vi "Device Manager.vi"() -> ()   [LabVIEW 2026]
doc: "This template is for the Queued Message Handler design pattern.\n\nThe Event Handling Loop generates messages based on user interface actions.\n\nThe Message Handling Loop processes messages generated by the Event Handling Loop, or by other messages. The messages are string values, so new messages can be added easily to the Message Cases case structure in the Message Handling Loop. Each message cluster can also provide an optional value for Message Data, which is a variant that can be converted to whatever message-specific data is required."
uses:
  controls/Device Manager Private Data.ctl
  support/Message Queue/Enqueue Message (Single).vi
  <vilib>/Utility/error.llb/Error Cluster From Error Code.vi
  <vilib>/ErrorRing/Error Ring.xnode
  support/Message Queue/Message Queue.lvlib
  support/User Event - Stop/User Event - Stop.lvlib
panel:
  in  "Exit":bool
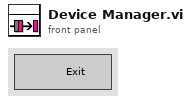
[diagram p1: front panel]
types:
  T1 = typedef "Device Manager Private Data.ctl" = cluster{"Exit Button Ref":refnum<vi>}
  T2 = typedef "Message Queue.lvlib/All Message Queues.ctl" = cluster{"Device Manager":refnum<queue>, "Front Panel Emulator":refnum<queue>, "Servo Motor Emulator":refnum<queue>}
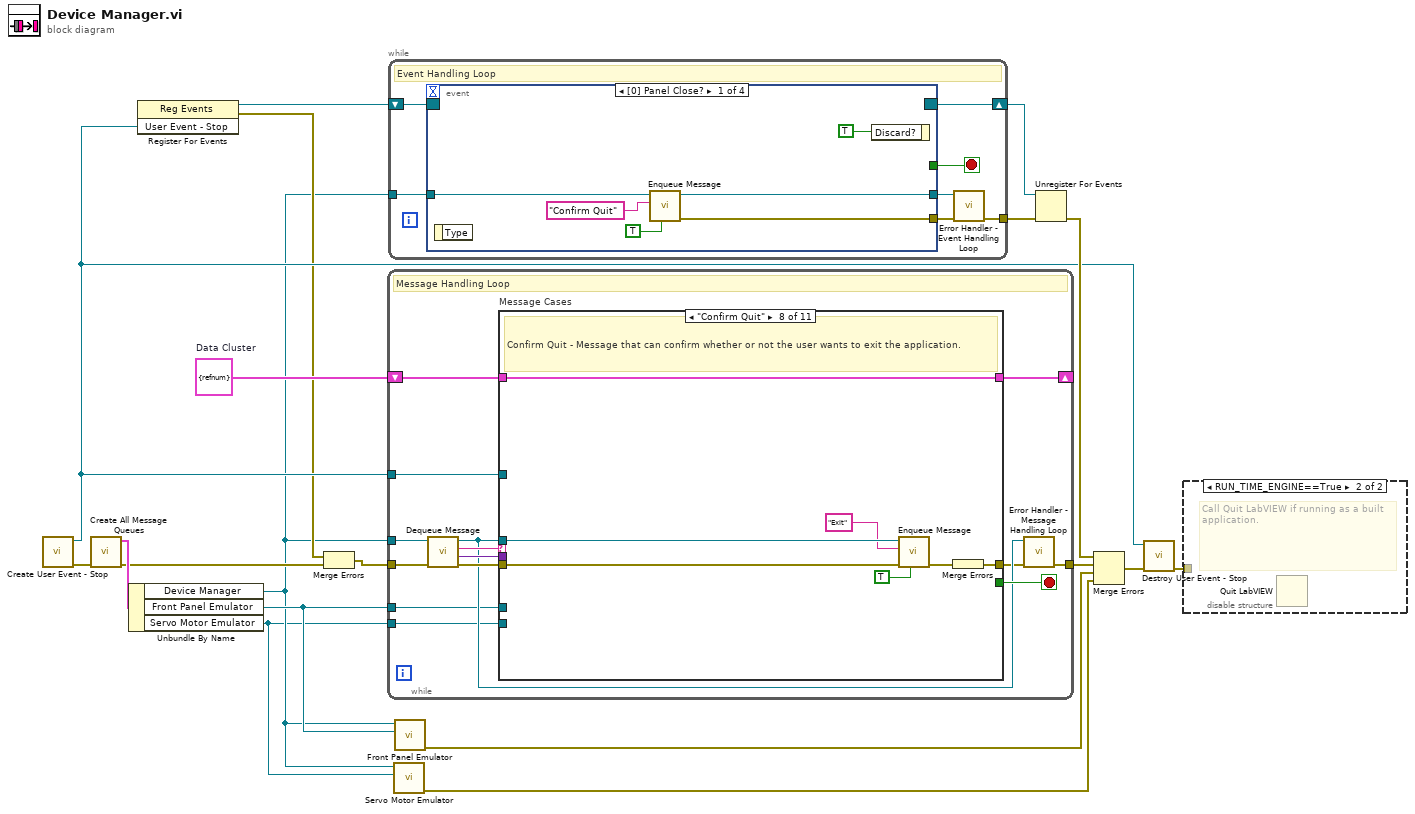
[diagram p0: block diagram]
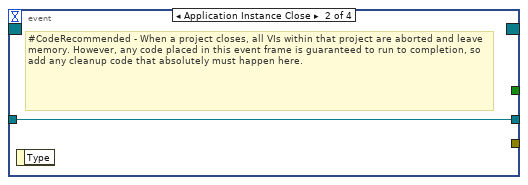
[diagram p3: hidden frame]
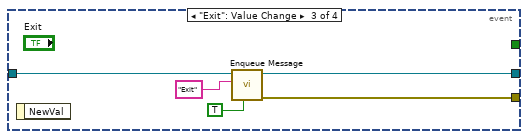
[diagram p4: hidden frame]
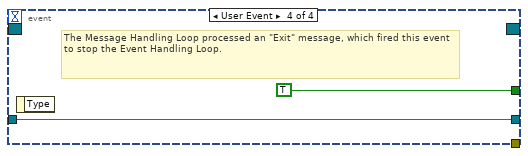
[diagram p5: hidden frame]
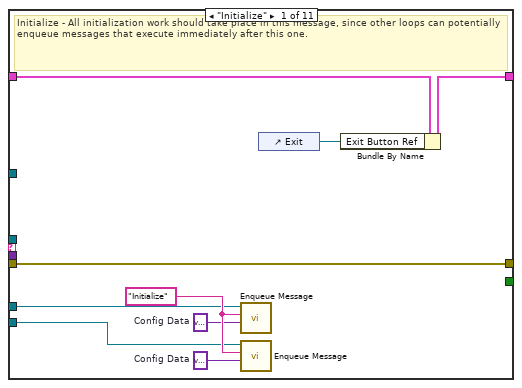
[diagram p6: hidden frame]
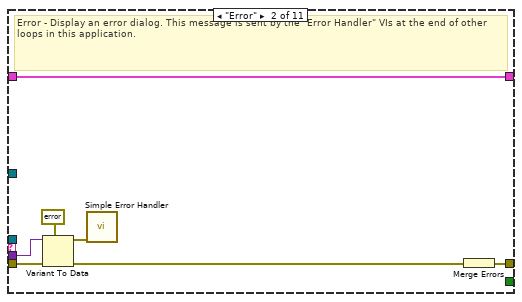
[diagram p7: hidden frame]
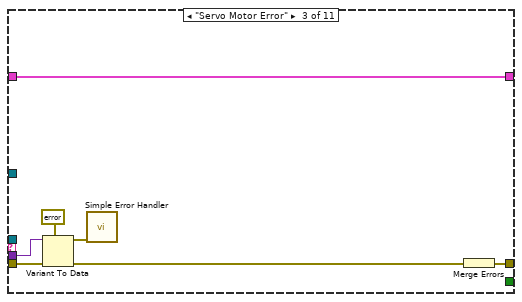
[diagram p8: hidden frame]
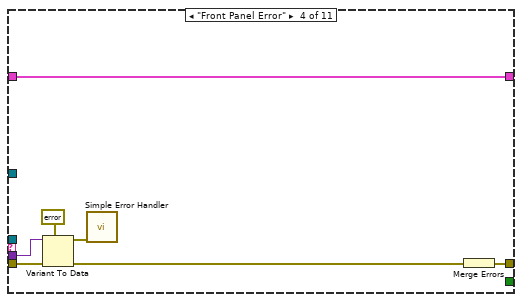
[diagram p9: hidden frame]
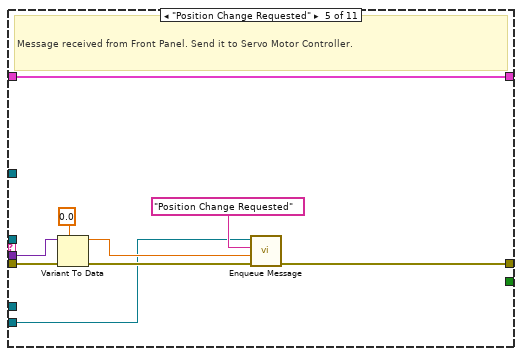
[diagram p10: hidden frame]
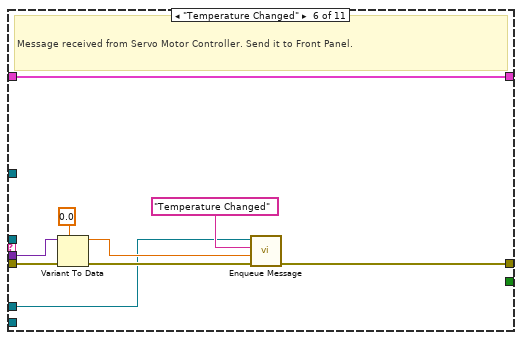
[diagram p11: hidden frame]
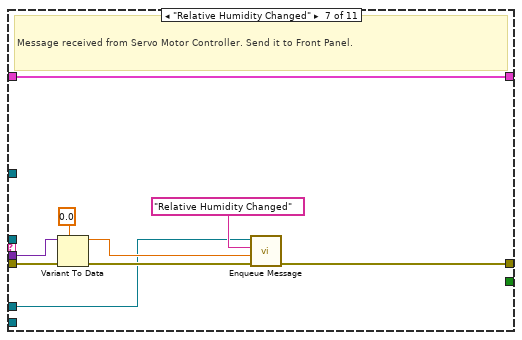
[diagram p12: hidden frame]
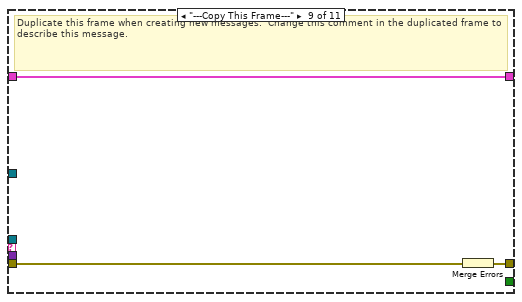
[diagram p13: hidden frame]
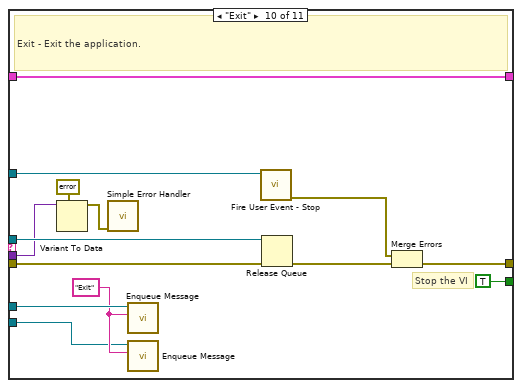
[diagram p14: hidden frame]
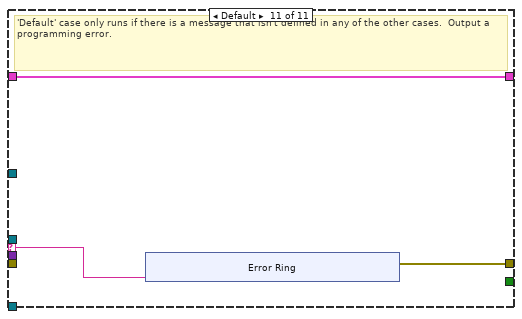
[diagram p15: hidden frame]
diagram:
  w13 = T1 {"Exit Button Ref"=refnum}  # Data Cluster
  n1 = call "Create User Event - Stop.vi"() -> ("error out"=w17:errorcluster, "User Event - Stop"=w9:refnum<user-event>)  [unwired: 10 in]
  n2 = call "Create All Message Queues.vi"("error in (no error)"=w17) -> ("error out"=w7:errorcluster, "Message Queues out"=w19:T2)  [unwired: 9 in]
  n3 = Unbundle By Name(w19) -> ("Device Manager"=w3:refnum<queue>, "Front Panel Emulator"=w4:refnum<queue>, "Servo Motor Emulator"=w2:refnum<queue>)
  n4 = register-events(w9) -> (reference out=w10:refnum<event-registration>, error out=w8:errorcluster)  [unwired: 2 in]
  n5 = Merge Errors(w8, w7) -> (w6:errorcluster)
  n6 = while {
    tunnel: w3 -> [w25]
    shift-right: [w32] -> _
    shift-left: w13 -> [w33]
    tunnel: w9 -> [w30]
    tunnel: w6 -> [w29]
    tunnel: [w23] -> w18
    tunnel: w4 -> [w21]
    tunnel: w2 -> [w20]
    stop <- w31 stop-if-true
    # "Message Handling Loop"
    n7 = call "Dequeue Message.vi"("error in (no error)"=w29, "Message Queue"=w25) -> ("error out"=w28:errorcluster, "Message Data"=w26:variant, "Message"=w27:string, "dup Message Queue"=w24:refnum<queue>)  [unwired: 6 in]
    n8 = case "Message Cases" shown="\"Confirm Quit\"" w27 {
      selector: w27 -> [_ _ _ _ _ _ _ _ _ _ w115]
      tunnel: w24 -> [_ _ _ _ _ _ _ w93 _ w114 _]
      tunnel: w28 -> [w34 w49 w56 w63 w66 w75 w84 w97 w100 w107 _]
      tunnel: [w34 w43 w50 w57 w67 w76 w85 w95 w98 w110 w116] -> w22
      tunnel: w33 -> [w42 w48 w55 w62 w72 w81 w90 w96 w99 w113 w117]
      tunnel: [w41 w48 w55 w62 w72 w81 w90 w96 w99 w113 w117] -> w32
      tunnel: [_ _ _ _ _ _ _ _ _ TRUE _] -> w31
      tunnel: w26 -> [_ w47 w54 w61 w65 w74 w83 _ _ w104 _]
      tunnel: w30 -> [_ _ _ _ _ _ _ _ _ w109 _]
      tunnel: w21 -> [w38 _ _ _ _ w73 w82 _ _ w103 _]
      tunnel: w20 -> [w37 _ _ _ w64 _ _ _ _ w101 _]
      frame "Initialize" {
        w35 = variant  # Config Data
        w36 = variant  # Config Data
        w39 = "Initialize" ("Message")
        # "Initialize - All initialization work should take place in this message, since other loops can potentially enqueue messages that execute immediately after this one."
        n9 = call-poly "Enqueue Message.vi"("Message Data"=w36, "Message"=w39, "Message Queue"=w38) -> ()  [unwired: 7 in, 2 out]
        n10 = call-poly "Enqueue Message.vi"("Message Data"=w35, "Message"=w39, "Message Queue"=w37) -> ()  [unwired: 7 in, 2 out]
        n11 = control-ref of="Exit"() -> (w40:refnum<vi>)
        n12 = Bundle By Name(cluster=w42, "Exit Button Ref"=w40) -> (w41:T1)
      }
      frame "Error" {
        # "Error - Display an error dialog. This message is sent by the \"Error Handler\" VIs at the end of other loops in this application."
        n13 = Variant To Data(error in=w49, type=errorcluster {"status"=FALSE, "code"=0, "source"=""} ("error constant"), Variant=w47) -> (data=w45:errorcluster, error out=w44:errorcluster)
        n14 = call <vilib>:"Simple Error Handler.vi"("error in (no error)"=w45) -> ()  [unwired: 4 in, 5 out]
        n15 = Merge Errors(w44) -> (w43:errorcluster)
      }
      frame "Servo Motor Error" {
        n16 = Variant To Data(error in=w56, type=errorcluster {"status"=FALSE, "code"=0, "source"=""} ("error constant"), Variant=w54) -> (data=w52:errorcluster, error out=w51:errorcluster)
        n17 = call <vilib>:"Simple Error Handler.vi"("error in (no error)"=w52) -> ()  [unwired: 4 in, 5 out]
        n18 = Merge Errors(w51) -> (w50:errorcluster)
      }
      frame "Front Panel Error" {
        n19 = Variant To Data(error in=w63, type=errorcluster {"status"=FALSE, "code"=0, "source"=""} ("error constant"), Variant=w61) -> (data=w59:errorcluster, error out=w58:errorcluster)
        n20 = call <vilib>:"Simple Error Handler.vi"("error in (no error)"=w59) -> ()  [unwired: 4 in, 5 out]
        n21 = Merge Errors(w58) -> (w57:errorcluster)
      }
      frame "Position Change Requested" {
        # "Message received from Front Panel. Send it to Servo Motor Controller."
        n22 = Variant To Data(error in=w66, type=0.0 ("Position"), Variant=w65) -> (data=w68:dbl, error out=w69:errorcluster)
        n23 = call-poly "Enqueue Message.vi"("error in (no error)"=w69, "Message Data"=w68, "Message"="Position Change Requested", "Message Queue"=w64) -> ("error out"=w67:errorcluster)  [unwired: 6 in, 1 out]
      }
      frame "Temperature Changed" {
        # "Message received from Servo Motor Controller. Send it to Front Panel."
        n24 = Variant To Data(error in=w75, type=0.0 ("Position"), Variant=w74) -> (data=w77:dbl, error out=w78:errorcluster)
        n25 = call-poly "Enqueue Message.vi"("error in (no error)"=w78, "Message Data"=w77, "Message"="Temperature Changed", "Message Queue"=w73) -> ("error out"=w76:errorcluster)  [unwired: 6 in, 1 out]
      }
      frame "Relative Humidity Changed" {
        # "Message received from Servo Motor Controller. Send it to Front Panel."
        n26 = Variant To Data(error in=w84, type=0.0 ("Position"), Variant=w83) -> (data=w86:dbl, error out=w87:errorcluster)
        n27 = call-poly "Enqueue Message.vi"("error in (no error)"=w87, "Message Data"=w86, "Message"="Relative Humidity Changed", "Message Queue"=w82) -> ("error out"=w85:errorcluster)  [unwired: 6 in, 1 out]
      }
      frame "Confirm Quit" {
        # "Confirm Quit - Message that can confirm whether or not the user wants to exit the application."
        n28 = call-poly "Enqueue Message.vi"("Priority Message? (F)"=TRUE, "error in (no error)"=w97, "Message"="Exit", "Message Queue"=w93) -> ("error out"=w94:errorcluster)  [unwired: 6 in, 1 out]
        n29 = Merge Errors(w94) -> (w95:errorcluster)
      }
      frame "---Copy This Frame---" {
        # "Duplicate this frame when creating new messages.  Change this comment in the duplicated frame to describe this message."
        n30 = Merge Errors(w100) -> (w98:errorcluster)
      }
      frame "Exit" {
        w102 = "Exit" ("Message")
        # "Stop the VI"
        # "Exit - Exit the application."
        n31 = Variant To Data(type=errorcluster {"status"=FALSE, "code"=0, "source"=""} ("error constant"), Variant=w104) -> (data=w105:errorcluster)  [unwired: 1 in, 1 out]
        n32 = call <vilib>:"Simple Error Handler.vi"("error in (no error)"=w105) -> ()  [unwired: 4 in, 5 out]
        n33 = call-poly "Enqueue Message.vi"("Message"=w102, "Message Queue"=w103) -> ()  [unwired: 8 in, 2 out]
        n34 = call-poly "Enqueue Message.vi"("Message"=w102, "Message Queue"=w101) -> ()  [unwired: 8 in, 2 out]
        n35 = call "Fire User Event - Stop.vi"("User Event - Stop"=w109) -> ("error out"=w108:errorcluster)  [unwired: 10 in]
        n36 = Release Queue(queue=w114, error in (no error)=w107) -> (error out=w111:errorcluster)  [unwired: 1 in, 2 out]
        n37 = Merge Errors(w108, w111) -> (w110:errorcluster)
      }
      frame Default {
        # "'Default' case only runs if there is a message that isn't defined in any of the other cases.  Output a programming error."
        n38 = xnode "Error Ring"("parameter 0"=w115) -> ("error out"=w116:errorcluster)
      }
    }
    n39 = call "Error Handler - Message Handling Loop.vi"("error in (no error)"=w22, "Message Queue"=w24) -> ("dup error in"=w23:errorcluster)  [unwired: 8 in, 1 out]
  }
  n40 = while {
    tunnel: w3 -> [w131]
    shift-right: [w129] -> w14
    shift-left: w10 -> [w130]
    tunnel: [w125] -> w11
    stop <- w127 stop-if-true
    # "Event Handling Loop"
    n41 = event shown="[0] Panel Close?" {
      selector: w130 -> [_ _ _ _]
      dyn-events: [_ _ _ _] -> w129
      timeout: _ -> [_ _ _ _]
      tunnel: [_ _ _ TRUE ("Discard?")] -> w127
      tunnel: w131 -> [w136 w138 w143 w145]
      tunnel: [w135 _ w142 _] -> w128
      tunnel: [w134 w138 w141 w145] -> w126
      event Panel Close? {
        n42 = event-data() -> ()  [unwired: 1 in, 1 out]
        n43 = call-poly "Enqueue Message.vi"("Priority Message? (F)"=TRUE, "Message"="Confirm Quit", "Message Queue"=w136) -> ("error out"=w135:errorcluster, "dup Message Queue"=w134:refnum<queue>)  [unwired: 7 in]
        n44 = event-data("Discard?"=TRUE) -> ()  [unwired: 1 in, 1 out]
      }
      event Application Instance Close {
        # "#CodeRecommended - When a project closes, all VIs within that project are aborted and leave memory. However, any code placed in this event frame is guaranteed to run to completion, so add any cleanup code that absolutely must happen here."
        n45 = event-data() -> ()  [unwired: 1 in, 1 out]
      }
      event "Exit": Value Change {
        n46 = event-data() -> ()  [unwired: 1 in, 1 out]
        n47 = call-poly "Enqueue Message.vi"("Priority Message? (F)"=TRUE, "Message"="Exit", "Message Queue"=w143) -> ("error out"=w142:errorcluster, "dup Message Queue"=w141:refnum<queue>)  [unwired: 7 in]
      }
      event User Event {
        # "The Message Handling Loop processed an \"Exit\" message, which fired this event to stop the Event Handling Loop."
        n48 = event-data() -> ()  [unwired: 1 in, 1 out]
      }
    }
    n49 = call "Error Handler - Event Handling Loop.vi"("error in (no error)"=w128, "Message Queue"=w126) -> ("dup error in"=w125:errorcluster)  [unwired: 8 in, 1 out]
  }
  n50 = call "Servo Motor Emulator.vi"("Servo Motor Emulator Queue in"=w2, "Device Manager Queue in"=w3) -> ("error out"=w1:errorcluster)  [unwired: 9 in]
  n51 = call "Front Panel Emulator.vi"("Front Panel Emulator Queue in"=w4, "Device Manager Queue in"=w3) -> ("error out"=w5:errorcluster)  [unwired: 9 in]
  n52 = Unregister For Events(event registration refnum=w14, error in=w11) -> (error out=w15:errorcluster)
  n53 = Merge Errors(w15, w18, w5, w1) -> (w16:errorcluster)
  n54 = call "Destroy User Event - Stop.vi"("error in (no error)"=w16, "User Event - Stop"=w9) -> ("error out"=w12:errorcluster)  [unwired: 9 in]
  n55 = disable-structure shown="RUN_TIME_ENGINE==True" {
    disable-tunnel: w12 -> [_ _]
    frame condition #0 (active) {
    }
    frame condition #1 {
      # "Call Quit LabVIEW if running as a built application."
      n56 = Quit LabVIEW() -> ()  [unwired: 1 in]
    }
  }
